vi "Clear.vi"(8 "error in (no error)":errorcluster, 11 "Low Level PSU In":refnum<class "Low Level PSU.lvclass">) -> (0 "error out":errorcluster, 3 "Low Level PSU Out":refnum<class "Low Level PSU.lvclass">)   [LabVIEW 2020, in "Low Level PSU With Tests.lvlib" / "Low Level PSU.lvclass"]
uses:
  Low Level PSU.lvclass
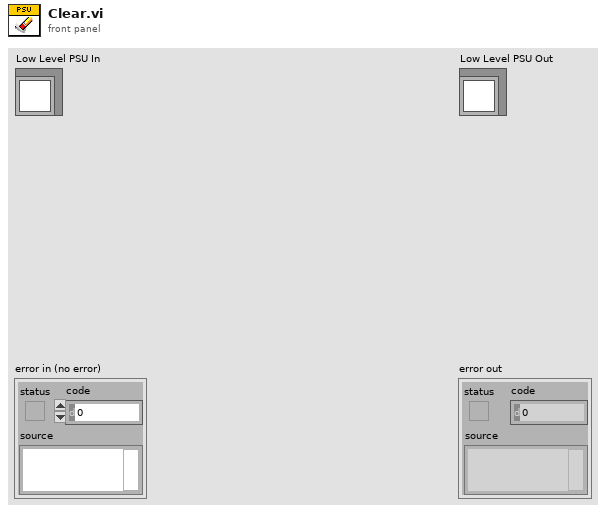
[diagram p1: front panel]
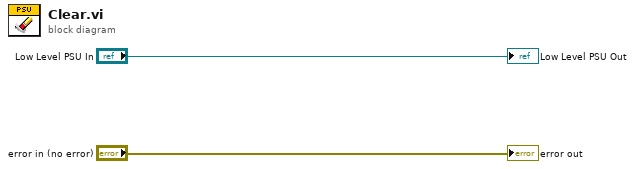
[diagram p0: block diagram]
diagram:
  "error out" <- "error in (no error)"
  "Low Level PSU Out" <- "Low Level PSU In"
